vi "Msg.vi"(7 "LVCAM in":refnum<class "LVCAM.lvclass">, 11 "LVCAM Nest Destroyed Msg in":refnum<class "LVCAM Nest Destroyed Msg.lvclass">) -> (0 "error out":errorcluster, 2 "Destroyed Self?":bool, 5 "LVCAM out":refnum<class "LVCAM.lvclass">)   [LabVIEW 2021, in "LVCAM Nest Destroyed.lvlib" / "LVCAM Nest Destroyed Msg.lvclass"]
uses:
  LVCAM Nest Destroyed Msg.lvclass
  LVCAM/LVCAM/LVCAM.lvclass
  LVCAM Nest Destroyed/LVCAM Nest Destroyed.lvclass
  LVCAM Nest Destroyed Msg.lvclass/LVCAM Nest Destroyed Msg.ctl
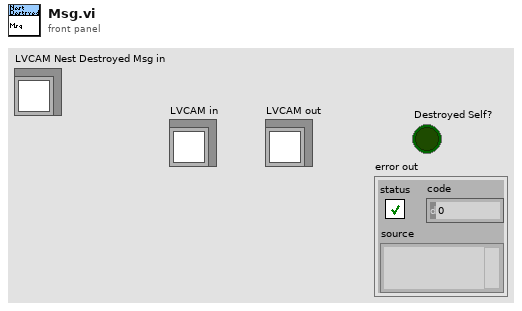
[diagram p1: front panel]
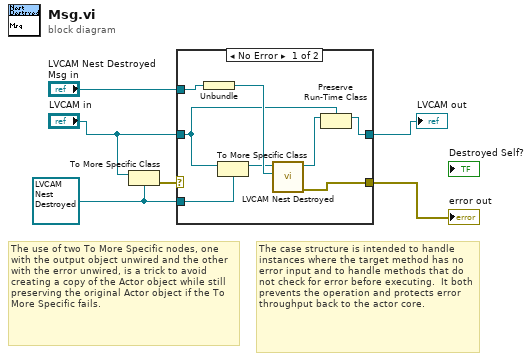
[diagram p0: block diagram]
diagram:
  w1 = refnum<class "LVCAM Nest Destroyed.lvclass"> refnum ("Last Ack.lvlib:Last Ack.lvclass")
  # "The use of two To More Specific nodes, one with the output object unwired and the other with the error unwired, is a trick to avoid creating a copy of the Actor object while still preserving the original Actor object if the To More Specific fails."
  # "The case structure is intended to handle instances where the target method has no error input and to handle methods that do not check for error before executing.  It both prevents the operation and protects error throughput back to the actor core."
  n1 = To More Specific Class(target class=w1, reference="LVCAM in") -> (error out=w6:errorcluster)  [unwired: 1 in, 1 out]
  n2 = case shown="No Error" w6 {
    selector: w6 -> [_ w16]
    tunnel: [w12 w16] -> w4
    tunnel: [w9 w15] -> w2
    tunnel: "LVCAM in" -> [w8 w15]
    tunnel: "LVCAM Nest Destroyed Msg in" -> [w14 _]
    tunnel: w1 -> [w7 _]
    frame No Error {
      n3 = Unbundle(w14) -> (w13:refnum<class "LVCAM.lvclass">)
      n4 = To More Specific Class(target class=w7, reference=w8) -> (specific class reference=w11:refnum<class "LVCAM Nest Destroyed.lvclass">)  [unwired: 1 in, 1 out]
      n5 = call-dynamic "LVCAM Nest Destroyed.vi"("Nest Actor"=w13, "LVCAM Nest Destroyed in"=w11) -> ("error out"=w12:errorcluster, "LVCAM Nest Destroyed out"=w10:refnum<class "LVCAM Nest Destroyed.lvclass">)  [unwired: 8 in]
      n6 = Preserve Run-Time Class(object in=w10, 2:w8) -> (object out=w9:refnum<class "LVCAM.lvclass">)  [unwired: 1 in, 1 out]
    }
    frame Error {
      # "If type check fails, pass the original object out again."
    }
  }
  "error out" <- w4
  "LVCAM out" <- w2
